vi "Bessel Polynomial.vi"(1 "n":u32, 2 "x":dbl format="%.2f") -> (0 "Bessel polynomial (n,x)":dbl format="%.2f")   [LabVIEW 2017, in "NI_Gmath.lvlib"]
doc: "Calculates the Bessel Polynomial of order <B>n</B> for any real number <B>x</B>."
uses:
  NI_Gmath.lvlib
  NI_AALBase.lvlib
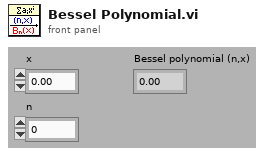
[diagram p1: front panel]
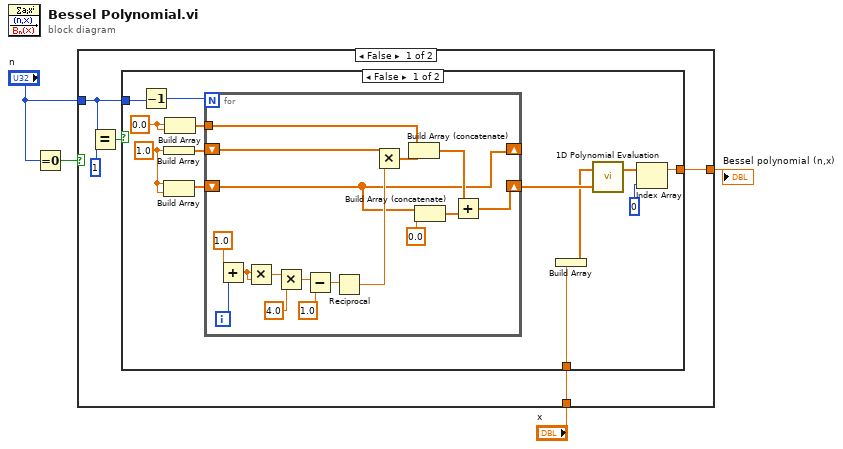
[diagram p0: block diagram]
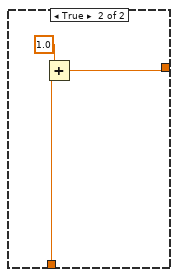
[diagram p2: hidden frame]
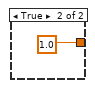
[diagram p3: hidden frame]
diagram:
  n1 = Equal To 0?(x="n") -> (x = 0?=w4:bool)
  n2 = case shown="False" w4 {
    tunnel: "n" -> [w6 _]
    tunnel: "x" -> [w8 _]
    tunnel: [w7 1.0] -> w2
    frame False {
      n3 = Equal?(x=w6, y=1) -> (x = y?=w9:bool)
      n4 = case shown="False" w9 {
        tunnel: w6 -> [w22 _]
        tunnel: w8 -> [w14 w42]
        tunnel: [w10 w40] -> w7
        frame False {
          w17 = 0.0
          w19 = 1.0
          n5 = Decrement(x=w22) -> (x-1=w21:u32)
          n6 = Build Array(w19) -> (w20:dbl[])
          n7 = Build Array(w19, w19) -> (w18:dbl[])
          n8 = Build Array(w17, w17) -> (w16:dbl[])
          n9 = for {
            N: w21 -> [_]
            shift-right: [w24] -> _
            shift-left: w20 -> [w29]
            shift-right: [w23] -> w15
            shift-left: w18 -> [w24]
            tunnel: w16 -> [w31]
            i -> [w39]
            n10 = Add(x=1.0, y=w39) -> (x+y=w37:dbl)
            n11 = Multiply(x=w37, y=w37) -> (x*y=w36:dbl)
            n12 = Multiply(x=w36, y=4.0) -> (x*y=w33:dbl)
            n13 = Subtract(x=w33, y=1.0) -> (x-y=w32:dbl)
            n14 = Reciprocal(x=w32) -> (1/x=w30:dbl)
            n15 = Multiply(x=w29, y=w30) -> (x*y=w28:dbl[])
            n16 = Build Array (concatenate)(w31, w28) -> (w26:dbl[])
            n17 = Build Array (concatenate)(w24, 0.0) -> (w25:dbl[])
            n18 = Add(x=w26, y=w25) -> (x+y=w23:dbl[])
          }
          n19 = Build Array(w14) -> (w13:dbl[])
          n20 = call "1D Polynomial Evaluation.vi"("Coefficients: a"=w15, "X"=w13) -> ("Y"=w12:dbl[])  [unwired: 1 out]
          n21 = Index Array(array=w12, index=0) -> (element=w10:dbl)
        }
        frame True {
          n22 = Add(x=1.0, y=w42) -> (x+y=w40:dbl)
        }
      }
    }
    frame True {
    }
  }
  "Bessel polynomial (n,x)" <- w2
